vi "Save Function FGV.vi"(7 "Channel Name in":string[](array[string]), 8 "error in":errorcluster, 9 "file path in":path, 10 "data in":dbl[](array[numeric]), 11 "CMD":T1(ring)) -> (0 "error out":errorcluster, 1 "file path out":path, 2 "Channel Name":string[](array[string]))   [LabVIEW 2018]
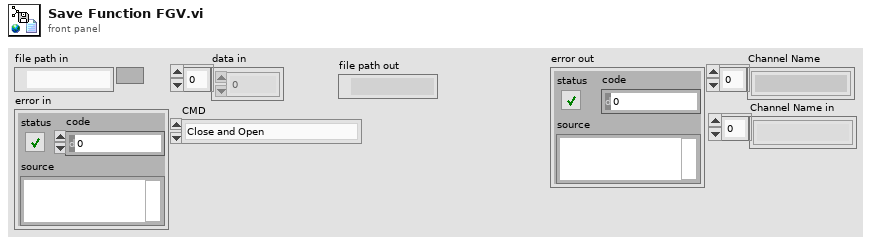
[diagram p1: front panel]
types:
  T1 = enum16{"Close and Open", "Write", "Write Header", "Close"}
  T2 = enum16{"open", "replace", "create", "open or create", "replace or create", "replace or create with confirmation"}
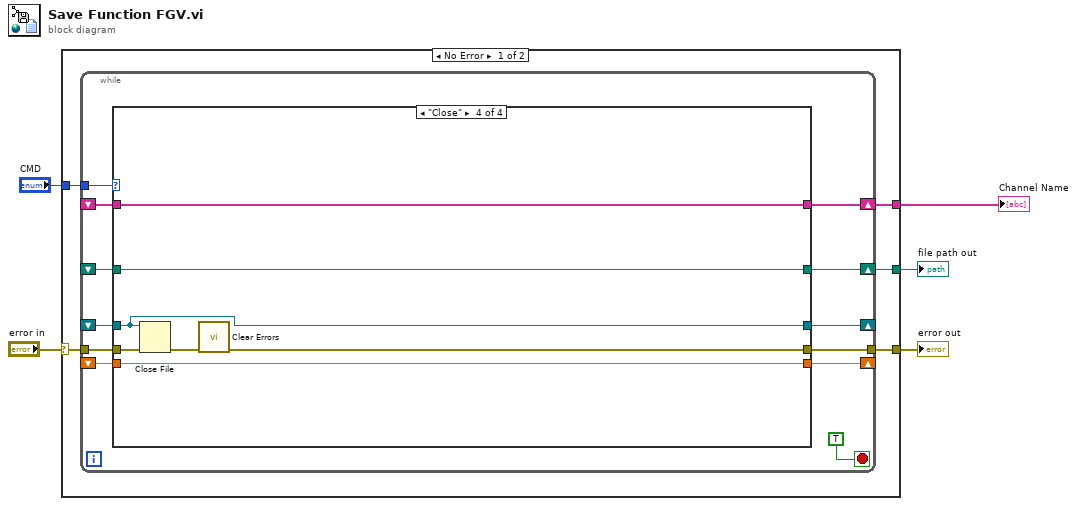
[diagram p0: block diagram]
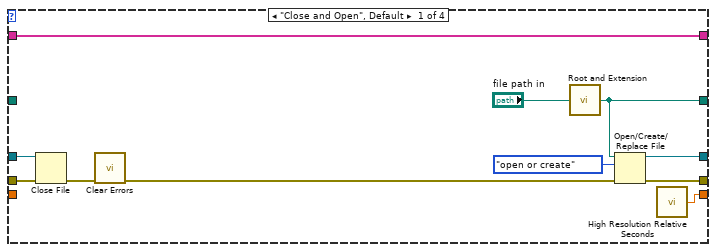
[diagram p2: hidden frame]
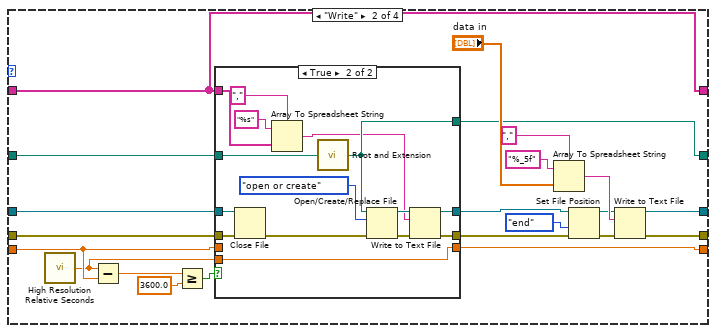
[diagram p3: hidden frame]
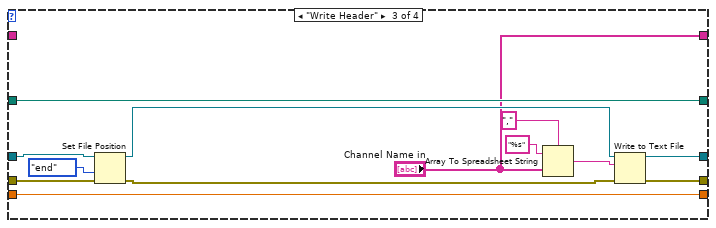
[diagram p5: hidden frame]
diagram:
  n1 = case shown="No Error" "error in" {
    selector: "error in" -> [w8 w95]
    tunnel: "CMD" -> [w10 _]
    tunnel: [w9 w95] -> w4
    tunnel: [w7 _] -> w2
    tunnel: [w6 _] -> w1
    frame No Error {
      n2 = while {
        tunnel: w10 -> [w21]
        shift-right: [w20] -> _
        shift-left: _ -> [w17]
        tunnel: [w19] -> w9
        tunnel: w8 -> [w18]
        shift-right: [w16] -> w7
        shift-left: _ -> [w15]
        shift-right: [w14] -> _
        shift-left: _ -> [w13]
        shift-right: [w12] -> w6
        shift-left: _ -> [w11]
        stop <- TRUE stop-if-true
        n3 = case shown="\"Close\"" w21 {
          tunnel: [w32 w54 w86 w92] -> w20
          tunnel: [w31 w55 w87 w91] -> w19
          tunnel: w18 -> [w29 w38 w78 w94]
          tunnel: w17 -> [w30 w40 w79 w92]
          tunnel: [w24 w35 w77 w90] -> w16
          tunnel: w15 -> [_ w36 w77 w90]
          tunnel: [w26 w42 w76 w89] -> w14
          tunnel: w13 -> [_ w43 w76 w89]
          tunnel: [w23 w34 "Channel Name in" w88] -> w12
          tunnel: w11 -> [w23 w34 _ w88]
          frame "Close and Open", Default {
            n4 = Close File(refnum=w30, error in=w29) -> (error out=w28:errorcluster)  [unwired: 1 out]
            n5 = call <vilib>:"Clear Errors.vi"("error in (no error)"=w28) -> ("error out"=w27:errorcluster)  [unwired: 5 in, 1 out]
            n6 = call "Root and Extension.vi"("File name in"="file path in") -> ("File name out"=w24:path)
            n7 = Open/Create/Replace File(file path (use dialog)=w24, error in=w27, operation (0:open)=T2."open or create") -> (refnum out=w32:refnum<file>, error out=w31:errorcluster)  [unwired: 3 in, 1 out]
            n8 = call <vilib>:"High Resolution Relative Seconds.vi"() -> ("relative seconds"=w26:dbl)
          }
          frame "Write" {
            n9 = call <vilib>:"High Resolution Relative Seconds.vi"() -> ("relative seconds"=w41:dbl)
            n10 = Subtract(x=w41, y=w43) -> (x-y=w46:dbl)
            n11 = Greater Or Equal?(x=w46, y=3600.0) -> (x >= y?=w44:bool)
            n12 = case shown="True" w44 {
              tunnel: [w59 w74] -> w42
              tunnel: w43 -> [w59 _]
              tunnel: w41 -> [_ w74]
              tunnel: w40 -> [w58 w73]
              tunnel: [w58 w64] -> w39
              tunnel: w38 -> [w57 w71]
              tunnel: [w57 w65] -> w37
              tunnel: w36 -> [w56 w70]
              tunnel: [w56 w69] -> w35
              tunnel: w34 -> [_ w61]
              frame False {
              }
              frame True {
                n13 = Close File(refnum=w73, error in=w71) -> (error out=w72:errorcluster)  [unwired: 1 out]
                n14 = Array To Spreadsheet String(delimiter (Tab)=",", array=w61, 3:"%s" ("format string")) -> (spreadsheet string=w60:string)
                n15 = call "Root and Extension.vi"("File name in"=w70) -> ("File name out"=w69:path)
                n16 = Open/Create/Replace File(file path (use dialog)=w69, error in=w72, operation (0:open)=T2."open or create") -> (refnum out=w67:refnum<file>, error out=w66:errorcluster)  [unwired: 3 in, 1 out]
                n17 = Write to Text File(file (use dialog)=w67, text=w60, error in=w66) -> (refnum out=w64:refnum<file>, error out=w65:errorcluster)  [unwired: 1 in, 1 out]
              }
            }
            n18 = Array To Spreadsheet String(delimiter (Tab)=",", array="data in", 3:"%_5f" ("format string")) -> (spreadsheet string=w52:string)
            n19 = Set File Position(refnum=w39, from (0:start)=enum16{"start", "end", "current"}."end", error in=w37) -> (refnum out=w49:refnum<file>, error out=w47:errorcluster)  [unwired: 1 in]
            n20 = Write to Text File(file (use dialog)=w49, text=w52, error in=w47) -> (refnum out=w54:refnum<file>, error out=w55:errorcluster)  [unwired: 1 in, 1 out]
          }
          frame "Write Header" {
            n21 = Set File Position(refnum=w79, from (0:start)=enum16{"start", "end", "current"}."end", error in=w78) -> (refnum out=w82:refnum<file>, error out=w80:errorcluster)  [unwired: 1 in]
            n22 = Array To Spreadsheet String(delimiter (Tab)=",", array="Channel Name in", 3:"%s" ("format string")) -> (spreadsheet string=w84:string)
            n23 = Write to Text File(file (use dialog)=w82, text=w84, error in=w80) -> (refnum out=w86:refnum<file>, error out=w87:errorcluster)  [unwired: 1 in, 1 out]
          }
          frame "Close" {
            n24 = Close File(refnum=w92, error in=w94) -> (error out=w93:errorcluster)  [unwired: 1 out]
            n25 = call <vilib>:"Clear Errors.vi"("error in (no error)"=w93) -> ("error out"=w91:errorcluster)  [unwired: 5 in, 1 out]
          }
        }
      }
    }
    frame Error {
    }
  }
  "error out" <- w4
  "file path out" <- w2
  "Channel Name" <- w1
